vi "Read Oxygen Signal Phase.vi"(0 "Session Handle in":T1, 11 "error in (no error)":errorcluster) -> (4 "Session Handle out":T1, 6 "Phase":dbl, 15 "error out":errorcluster)   [LabVIEW 2015, in "Gas.lvclass"]
uses:
  Gas.lvclass
  Typedefs/Session Handle.ctl
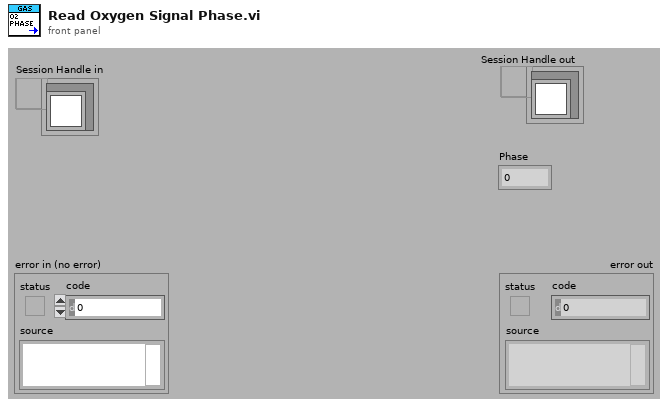
[diagram p1: front panel]
types:
  T1 = typedef "Gas.lvclass/Session Handle.ctl" = refnum<data-value>
  T2 = typedef "XNET Frame CAN.ctl" = cluster{"timestamp":timestamp, "payload":u8[], "identifier":u32, "type":T3, "extended?":bool, "echo?":bool}
  T3 = typedef "XNET Frame Type CAN.ctl" = u8
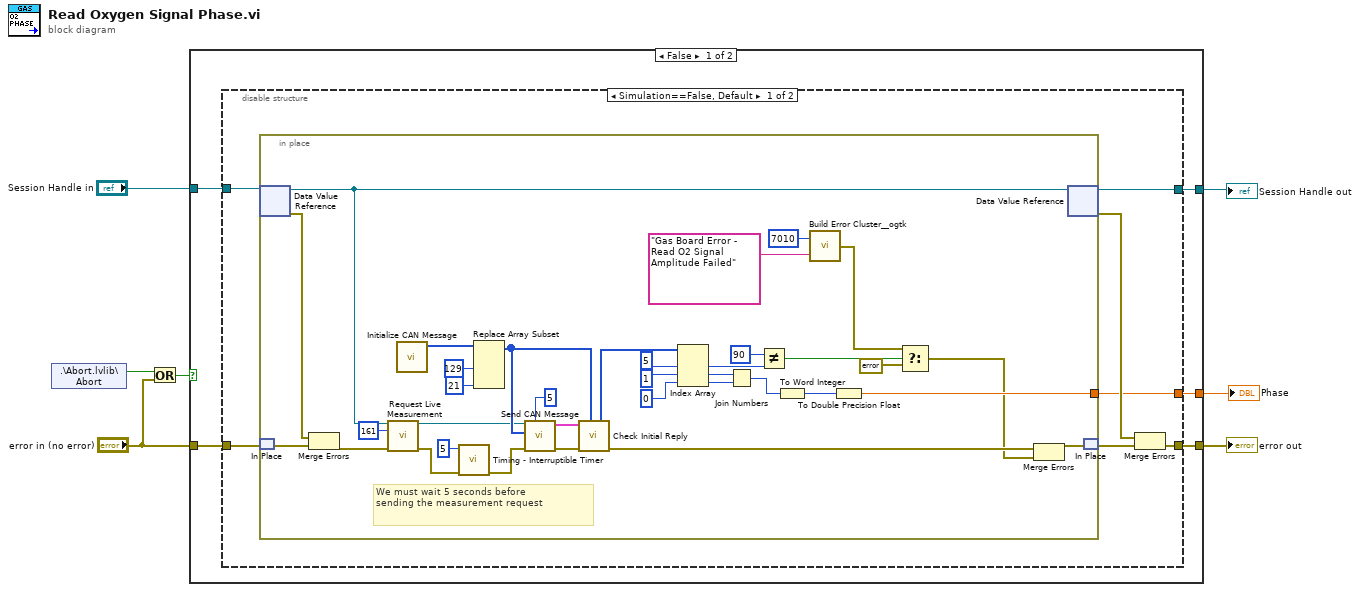
[diagram p0: block diagram]
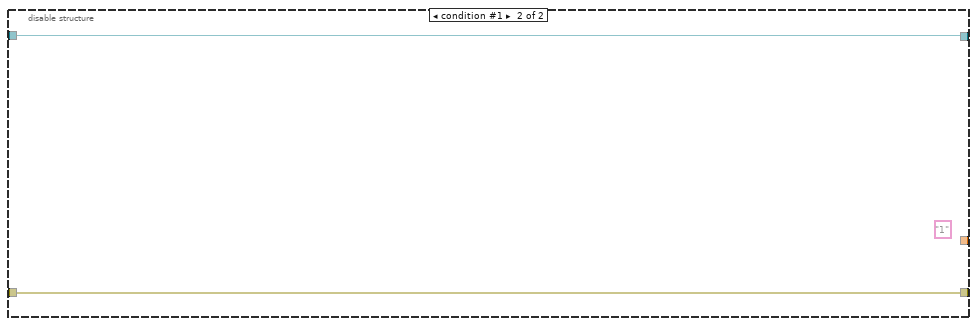
[diagram p2: hidden frame]
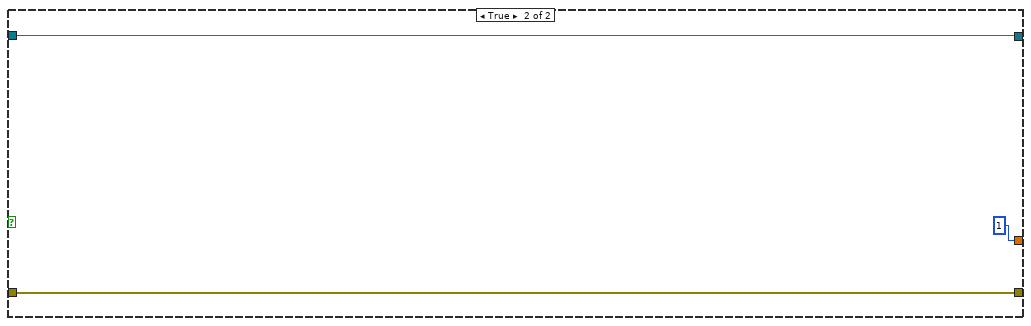
[diagram p3: hidden frame]
diagram:
  n1 = shared-variable ".\\Abort.lvlib\\Abort"() -> (w4:bool)  [unwired: 1 in, 1 out]
  n2 = Or(x=w4, y="error in (no error)") -> (x .or. y?=w2:bool)
  n3 = case shown="False" w2 {
    tunnel: [w12 w59] -> w6
    tunnel: [w11 w58] -> w5
    tunnel: "Session Handle in" -> [w10 w59]
    tunnel: "error in (no error)" -> [w9 w58]
    tunnel: [w8 u16 1] -> w1
    frame False {
      n4 = disable-structure shown="Simulation==False, Default" {
        disable-tunnel: [w19 w56] -> w12
        disable-tunnel: [w16 w55] -> w11
        disable-tunnel: w10 -> [w15 w56]
        disable-tunnel: w9 -> [w14 w55]
        disable-tunnel: [w13 _] -> w8
        frame condition #0 (active) {
          n5 = in-place {
            in-place-border: [w23] -> w13
            # "We must wait 5 seconds before \nsending the measurement request"
            n6 = in-place-dvr #1(w15) -> (w34:refnum<class "Gas.lvclass">, w49:errorcluster)
            n7 = in-place-match #2(w14) -> (w48:errorcluster)
            n8 = Merge Errors(w49, w48) -> (w35:errorcluster)
            n9 = call "Request Live Measurement.vi"("Gas In"=w34, "Request Type"=u8 161, "error in (no error)"=w35) -> ("Gas Out"=w31:refnum<class "Gas.lvclass">, "error out"=w32:errorcluster)  [unwired: 10 in, 1 out]
            n10 = call "Initialize CAN Message.vi"() -> ("Initial Payload"=w51:u8[])  [unwired: 11 in]
            n11 = call "Timing - Interruptible Timer.vi"("error in (no error)"=w32, "Wait (s)"=5) -> ("error out"=w30:errorcluster)  [unwired: 7 in, 2 out]
            n12 = Replace Array Subset(array=w51, new element #1=u8 129 ("new element/subarray"), new element #2=u8 21 ("new element/subarray")) -> (w47:u8[])  [unwired: 2 in]
            n13 = call "Send CAN Message.vi"("Number of Retries"=5, "error in (no error)"=w30, "payload"=w47, "Gas In"=w31) -> ("error out"=w22:errorcluster, "Reply"=w45:T2[])  [unwired: 5 in, 1 out]
            n14 = call "Check Initial Reply.vi"("Write Message"=w47, "error in (no error)"=w22, "Reply"=w45) -> ("error out"=w21:errorcluster, "Data Packet"=w50:u8[])  [unwired: 5 in, 2 out]
            n15 = Index Array(array=w50, index #1=5 ("index"), index #2=1 ("index"), index #3=0 ("index")) -> (element #1=w39:u8, element #2=w27:u8, element #3=w26:u8)
            n16 = Join Numbers(hi=w27, lo=w26) -> ((hi.lo)=w24:u16)
            n17 = Not Equal?(x=u8 90 ("new element/subarray"), y=w39) -> (x != y?=w37:bool)
            n18 = To Word Integer(number=w24) -> (16bit integer=w25:i16)
            n19 = call <userlib>:"Build Error Cluster__ogtk.vi"("String to Prepend to source (\"\")"="Gas Board Error - Read O2 Signal Amplitude Failed" ("string"), "code"=7010) -> ("error out"=w42:errorcluster)
            n20 = To Double Precision Float(number=w25) -> (double precision float=w23:dbl)
            n21 = Select(t=w42, s=w37, f=errorcluster {"status"=FALSE, "code"=0, "source"=""}) -> (s? t:f=w20:errorcluster)
            n22 = Merge Errors(w21, w20) -> (w52:errorcluster)
            n23 = in-place-dvr #1(w34) -> (w19:T1, w17:errorcluster)
            n24 = in-place-match #2(w52) -> (w18:errorcluster)
          }
          n25 = Merge Errors(w17, w18) -> (w16:errorcluster)
        }
        frame condition #1 {
          (unwired) "1"
        }
      }
    }
    frame True {
    }
  }
  "Session Handle out" <- w6
  "error out" <- w5
  "Phase" <- w1
